vi "FPGA_Slave_v01.vi"() -> ()   [LabVIEW 2014]
uses:
  <vilib>/Platform/TimedLoop/XDataNode/timing_clust.ctl
  <vilib>/Platform/TimedLoop/XDataNode/nitl_modes.ctl
  <vilib>/Platform/TimedLoop/XDataNode/wakeup.ctl
  <vilib>/rvi/Emulation/niFpgaGetClockAttributes.vi
  <vilib>/rvi/Emulation/niFpgaSctlEmulationGetInTimedLoop.vi
  <vilib>/rvi/Emulation/niFpgaEmulationReportErrorSimple.vi
  <vilib>/rvi/eio/common/nirviEmuTemplateMethod_errors.vi
  <vilib>/rvi/Emulation/niFpgaCriticalErrorInLSC.vi
  <vilib>/eio/EIONode/EIONode.xnode
  <vilib>/Platform/TimedLoop/XDataNode/XDataNode.xnode
  <vilib>/Platform/TimedLoop/XDataNode/XDNodeRunTimeDep.lvlib
panel:
  in  "Furnace Power":fxp<+/-,20,5>
  in  "Heat Exch Fan":fxp<+/-,20,5>
  in  "Extract Fan Out":fxp<+/-,20,5>
  out "O2Data":T1
  in  "O2Control":T2
  in  "Fan Voltage Out":fxp<+/-,20,5>
  out "Expansion Input Array":fxp<+/-,34,9>[](array[numeric])
  out "error out":errorcluster
  # "OMEGA Expansion Chasis FPGA v01"
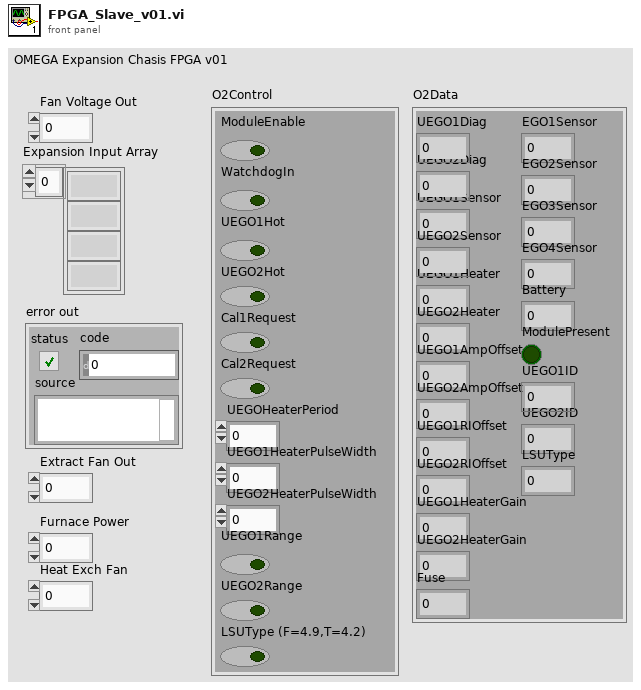
[diagram p1: front panel]
types:
  T1 = cluster{"UEGO1Diag":u8, "UEGO2Diag":u8, "UEGO1Sensor":u16, "UEGO2Sensor":u16, "UEGO1Heater":u16, "UEGO2Heater":u16, "UEGO1AmpOffset":u16, "UEGO2AmpOffset":u16, "UEGO1RIOffset":u16, "UEGO2RIOffset":u16, "UEGO1HeaterGain":u16, "UEGO2HeaterGain":u16, "Fuse":u16, "EGO1Sensor":u16, "EGO2Sensor":u16, "EGO3Sensor":u16, "EGO4Sensor":u16, "Battery":u16, "ModulePresent":bool, "UEGO1ID":u8, "UEGO2ID":u8, "LSUType":u8}
  T2 = cluster{"ModuleEnable":bool, "WatchdogIn":bool, "UEGO1Hot":bool, "UEGO2Hot":bool, "Cal1Request":bool, "Cal2Request":bool, "UEGOHeaterPeriod":u16, "UEGO1HeaterPulseWidth":u16, "UEGO2HeaterPulseWidth":u16, "UEGO1Range":bool, "UEGO2Range":bool, "LSUType (F=4.9,T=4.2)":bool}
  T3 = typedef "XDNodeRunTimeDep.lvlib/timing_clust.ctl" = cluster{"Expected End [f-1]":u64, "Actual End [f-1]":u64, "Finished Late? [f-1]":bool, "Expected End [i-1]":u64, "Actual End [i-1]":u64, "Finished Late? [i-1]":bool, "Expected Start [i]":u64, "Actual Start [i]":u64, "Expected Start [f]":u64, "Actual Start [f]":u64, "Source Name":string, "Structure Name":string, "Period":i64, "Deadline":i64, "Offset":i64, "Start":i64, "Priority":i32, "Timeout":i32, "Mode":T4, "Wakeup Reason":T5, "Error":errorcluster, "Source Type":string, "Secondary Source Type":string, "Global End Time":u64, "Global Start Time":u64, "Frame Duration":u64, "Iteration Duration":u64, "Assigned CPU":i32, "I/O Scan Engine Mode":u32}
  T4 = typedef "XDNodeRunTimeDep.lvlib/nitl_modes.ctl" = enum32{"No Change", "Process missed periods, maintain original phase", "Discard missed periods, maintain original phase", "Process missed periods, ignore original phase", "Discard missed periods, ignore original phase"}
  T5 = typedef "XDNodeRunTimeDep.lvlib/wakeup.ctl" = enum32{"Normal", "Aborted", "Asynchronous wakeup", "Timing source error", "Timed loop error", "Timeout"}
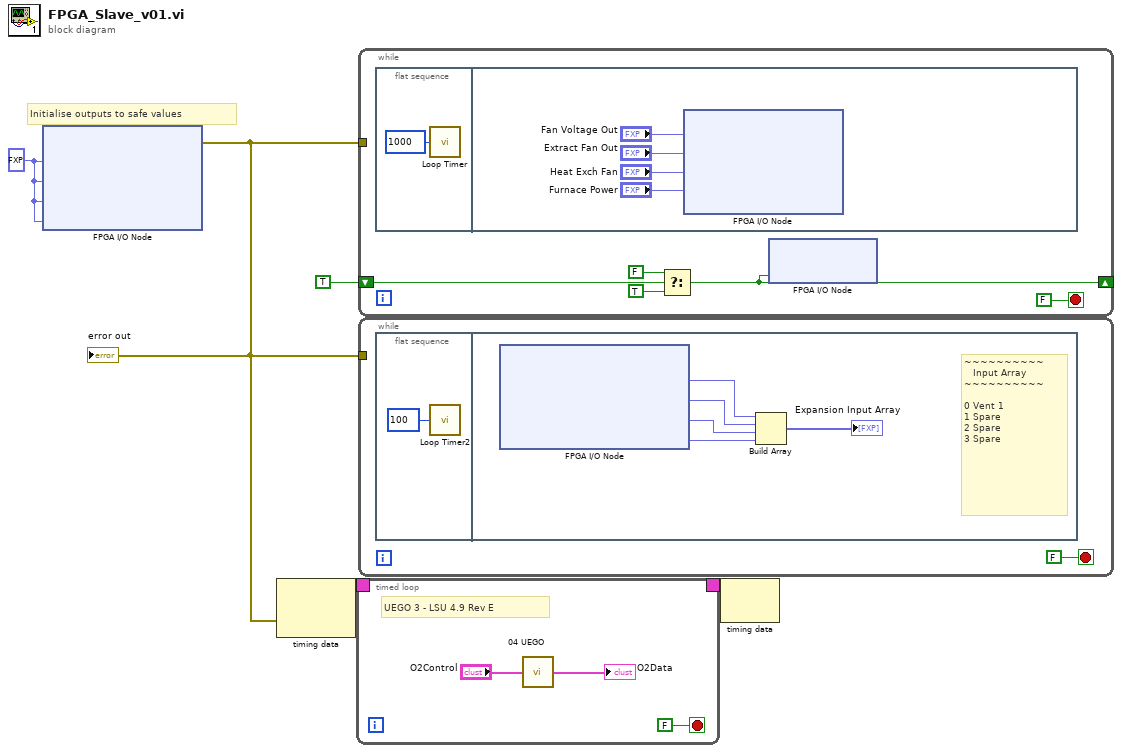
[diagram p0: block diagram]
diagram:
  w1 = fxp<+/-,20,5> 0.0 ("Inverter Fan 1")
  # "Initialise outputs to safe values"
  n1 = xnode "FPGA I/O Node"("01 Inverter_1"=w1, "02 Extractor Fan"=w1, "03 Heat Exch Fan"=w1, "04 Furnace Power"=w1) -> ("error out"=w2:errorcluster)  [unwired: 5 in, 4 out]
  "error out" <- w2
  n2 = node-c288(w2) -> (w4:T3)  [unwired: 1 in]
  n3 = timed-loop {
    timing: w4 -> [_]
    timing-out: [_] -> w3
    stop <- FALSE stop-if-true
    # "UEGO 3 - LSU 4.9 Rev E"
    n4 = call "04 UEGO"("O2Control"="O2Control") -> ("O2Data"=→"O2Data":T1)
  }
  n5 = while {
    tunnel: w2 -> [_]
    shift-right: [w11] -> _
    shift-left: TRUE -> [w14]
    stop <- FALSE stop-if-true
    n6 = flat-sequence {
      frame #0 {
        n7 = call "Loop Timer"("Count(mSec)"=u32 1000) -> ()  [unwired: 1 out]
      }
      frame #1 {
        n8 = xnode "FPGA I/O Node"("01 Inverter_1"="Fan Voltage Out", "02 Extractor Fan"="Extract Fan Out", "03 Heat Exch Fan"="Heat Exch Fan", "04 Furnace Power"="Furnace Power") -> ()  [unwired: 4 in, 4 out]
      }
    }
    n9 = Select(t=FALSE, s=w14, f=TRUE) -> (s? t:f=w11:bool)
    n10 = xnode "FPGA I/O Node"("FPGA LED"=w11) -> ()  [unwired: 1 in, 1 out]
  }
  n11 = while {
    tunnel: w2 -> [_]
    stop <- FALSE stop-if-true
    n12 = flat-sequence {
      frame #0 {
        n13 = call "Loop Timer2"("Count(mSec)"=u32 100) -> ()  [unwired: 1 out]
      }
      frame #1 {
        # "~~~~~~~~~~\n   Input Array\n~~~~~~~~~~\n\n0 Vent 1\n1 Spare\n2 Spare\n3 Spare"
        n14 = xnode "FPGA I/O Node"() -> ("Pressure_Transducer-1"=w25:fxp<+/-,21,-4>, "Pressure_Transducer-2"=w27:fxp<+/-,21,-4>, "Pressure_Transducer-3"=w24:fxp<+/-,21,-4>, "Pressure_Transducer-4"=w23:fxp<+/-,21,-4>)  [unwired: 5 in, 5 out]
        n15 = Build Array(w25, w27, w24, w23) -> (→"Expansion Input Array":fxp<+/-,21,-4>[])
      }
    }
  }
  n16 = node-c288(w3) -> ()  [unwired: 1 out]
